vi "calibrationElectrometer_putSample_loopTime.vi"(8 "error in (no error)":errorcluster, 11 "loopTime_Ctl":T1={"loopTime"=0.0, "electId"="                                                                                                                                                                                                                                                                "}) -> (0 "error out":errorcluster, 2 "function return":i32, 3 "loopTime_Ctl out":T1={"loopTime"=0.0, "electId"="                                                                                                                                                                                                                                                                "})   [LabVIEW 2016, in "SALLV_calibrationElectrometer.lvlib"]
doc: "int calibrationElectrometer_shm_putSample_loopTimeLV(calibrationElectrometer_loopTimeLV *loopTime_Ctl );"
uses:
  SALLV_calibrationElectrometer.lvlib
  DataTypes/loopTime.ctl
  SALLV_calibrationElectrometer.so
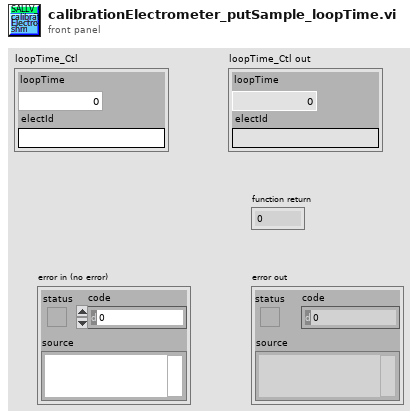
[diagram p1: front panel]
types:
  T1 = typedef "SALLV_calibrationElectrometer.lvlib/loopTime.ctl" = cluster{"loopTime":dbl, "electId":string}
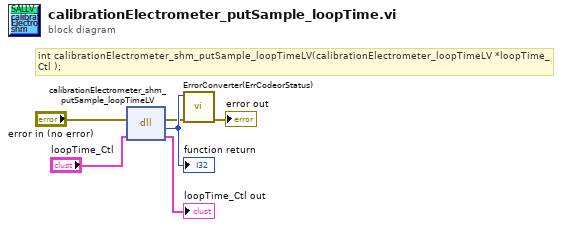
[diagram p0: block diagram]
diagram:
  # "int calibrationElectrometer_shm_putSample_loopTimeLV(calibrationElectrometer_loopTimeLV *loopTime_Ctl );"
  n1 = dll-call lib="home/andres/Desktop/SAL_calibrationElectrometer/SALLV_calibrationElectrometer.*" fn="calibrationElectrometer_shm_putSample_loopTimeLV"(error in="error in (no error)", "loopTime_Ctl"="loopTime_Ctl") -> (error out=w2:errorcluster, w6:i32, "loopTime_Ctl"=→"loopTime_Ctl out":T1)  [unwired: 2 in, 1 out]
  "function return" <- w6
  n2 = call "ErrorConverter(ErrCodeorStatus).vi"("error in (no error)"=w2, "error code"=w6) -> ("error out"=→"error out":errorcluster)  [unwired: 9 in]
